vi "Drop and wire SubVI.vi"(7 "Active VI Refnum":refnum<vi>, 8 "error in":errorcluster, 9 "BBN Node":refnum<vi>, 11 "Stub VI":refnum<vi>) -> (0 "error out":errorcluster, 1 "SubVI Output Terminal":refnum<vi>, 3 "SubVI":refnum<vi>)   [LabVIEW 2012, in "Build Cluster of References__RCF.lvlib"]
uses:
  Build Cluster of References__RCF.lvlib
  <vilib>/Utility/miscctls.llb/LVPointTypeDef.ctl
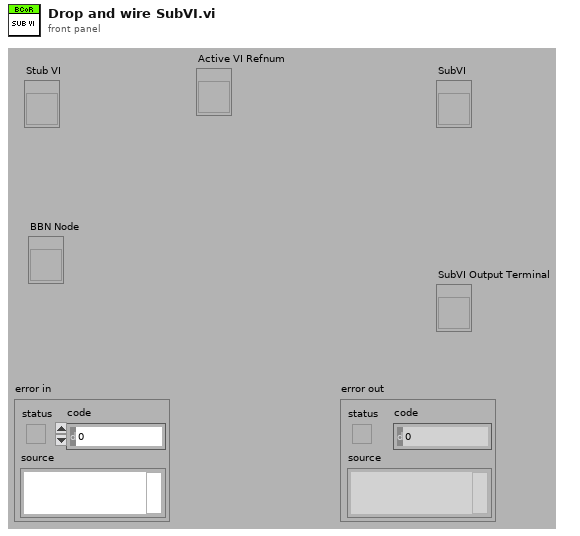
[diagram p1: front panel]
types:
  T1 = typedef "LVPointTypeDef.ctl" = cluster{"Horizontal":i16, "Vertical":i16}
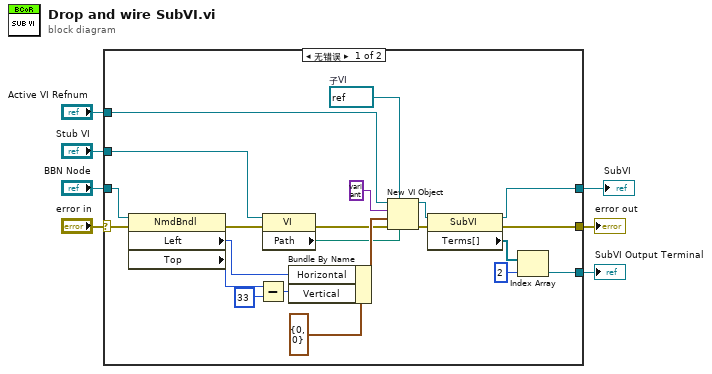
[diagram p0: block diagram]
diagram:
  n1 = case shown="无错误" "error in" {
    selector: "error in" -> [w13 w30]
    tunnel: [w29 _] -> w7
    tunnel: "Active VI Refnum" -> [w20 _]
    tunnel: "Stub VI" -> [w18 _]
    tunnel: "BBN Node" -> [w16 _]
    tunnel: [w9 w30] -> w3
    tunnel: [w8 _] -> w1
    frame No Error {
      w17 = refnum<vi> refnum  # 子VI
      n2 = property class="NmdBndl"(reference=w16, error in=w13) -> (error out=w12:errorcluster, "Left"=w15:i32, "Top"=w14:i32)  [unwired: 1 out]
      n3 = Subtract(x=w14, y=33) -> (x-y=w24:i32)
      n4 = property class="VI"(reference=w18, error in=w12) -> (error out=w11:errorcluster, "Path"=w19:path)  [unwired: 1 out]
      n5 = Bundle By Name(cluster=T1 {"Horizontal"=0, "Vertical"=0} ("relative position/next to refnum"), "Horizontal"=w15, "Vertical"=w24) -> (w23:T1)
      n6 = New VI Object(vi object class=w17, owner refnum=w20, style=variant, position/next to=w23, 6:w19, 8:w11) -> (object refnum=w26:refnum<vi>, 0:w10:errorcluster)  [unwired: 2 out]
      n7 = property class="SubVI"(reference=w26, error in=w10) -> (reference out=w8:refnum<vi>, error out=w9:errorcluster, "Terms[]"=w27:refnum<vi>[])
      n8 = Index Array(array=w27, index=2) -> (element=w29:refnum<vi>)
    }
    frame Error {
    }
  }
  "SubVI Output Terminal" <- w7
  "error out" <- w3
  "SubVI" <- w1
